vi "AddObject.vi"(1 "remote object ref":refnum<class "G#Object.lvclass">, 2 "proxy object ref":refnum<class "G#RemoteProxy.lvclass">, 3 "proxy class object ref":refnum<class "G#RemoteProxy.lvclass">, 5 "error in (no error)":errorcluster, 6 "full class name":string) -> (19 "error out":errorcluster)   [LabVIEW 2017, in "G#RemoteProxy.lvclass"]
doc: "Adds object to the local cache."
uses:
  G#RemoteProxy.lvclass
  G#Object/G#Object.lvclass
  C:/Program Files (x86)/National Instruments/LabVIEW 2017/vi.lib/addons/_AddQ/G#Object/G#Object.lvclass
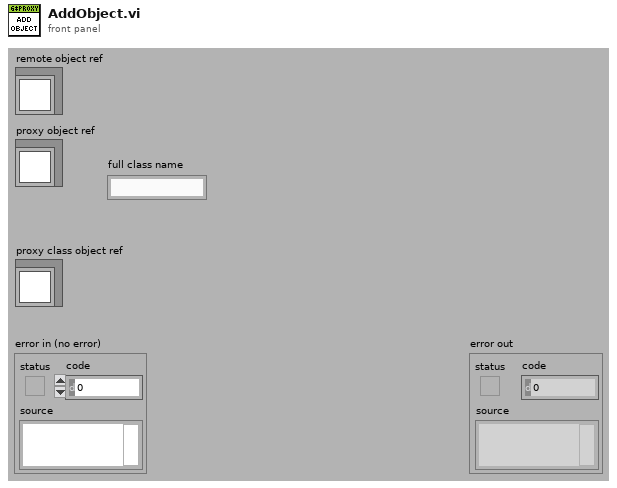
[diagram p1: front panel]
types:
  T1 = typedef "G#RemoteProxy.lvclass/ClassAttributesRef.ctl" = refnum<data-value>
  T2 = typedef "G#RemoteProxy.lvclass/ClassAttributesProxy.ctl" = cluster{"NoActiveProject":bool, "FullClassNames":string[], "FullClassPaths":path[], "RemoteRefs":refnum<class "G#Object.lvclass">[], "ProxyRefs":refnum<class "G#RemoteProxy.lvclass">[], "RemoteClassName":string[], "ProxyClassRefs":refnum<class "G#RemoteProxy.lvclass">[]}
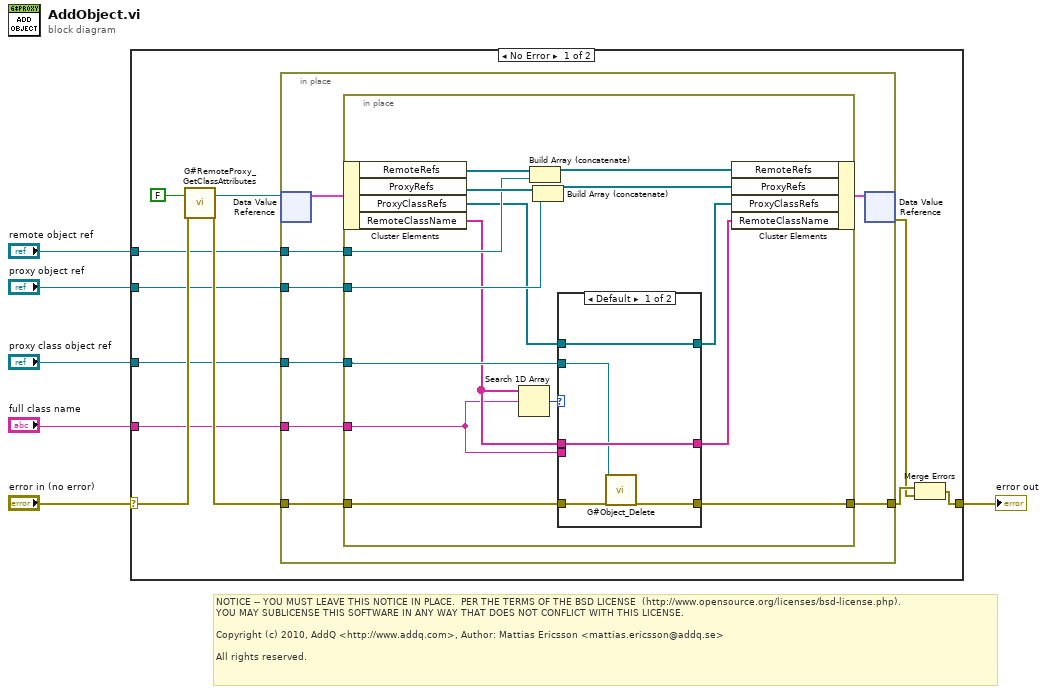
[diagram p0: block diagram]
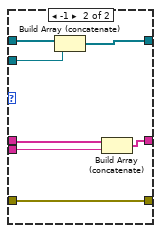
[diagram p2: hidden frame]
diagram:
  # "NOTICE -- YOU MUST LEAVE THIS NOTICE IN PLACE.  PER THE TERMS OF THE BSD LICENSE  (http://www.opensource.org/licenses/bsd-license.php).\nYOU MAY SUBLICENSE THIS SOFTWARE IN ANY WAY THAT DOES NOT CONFLICT WITH THIS LICENSE.\n\nCopyright (c) 2010, AddQ <http://www.addq.com>, Author: Mattias Ericsson <mattias.ericsson@addq.se>\n\nAll rights reserved."
  n1 = case shown="No Error" "error in (no error)" {
    selector: "error in (no error)" -> [w17 w53]
    tunnel: [w14 w53] -> w5
    tunnel: "remote object ref" -> [w10 _]
    tunnel: "proxy object ref" -> [w9 _]
    tunnel: "full class name" -> [w8 _]
    tunnel: "proxy class object ref" -> [w7 _]
    frame No Error {
      n2 = call "G#RemoteProxy_GetClassAttributes.vi"("return data? (T)"=FALSE ("return data"), "error in (no error)"=w17) -> ("class attributes ref"=w15:T1, "error out"=w16:errorcluster)  [unwired: 14 in, 2 out]
      n3 = in-place {
        in-place-border: w16 -> [w20]
        in-place-border: [w19] -> w12
        in-place-border: w10 -> [w23]
        in-place-border: w9 -> [w22]
        in-place-border: w8 -> [w21]
        in-place-border: w7 -> [w18]
        n4 = in-place-dvr #1(w15) -> (w24:T2)  [unwired: 1 out]
        n5 = in-place {
          in-place-border: w23 -> [w33]
          in-place-border: w22 -> [w36]
          in-place-border: w21 -> [w26]
          in-place-border: w20 -> [w34]
          in-place-border: [w29] -> w19
          in-place-border: w18 -> [w32]
          n6 = in-place-cluster #2(w24) -> ("RemoteRefs"=w40:refnum<class "G#Object.lvclass">[], "ProxyRefs"=w37:refnum<class "G#RemoteProxy.lvclass">[], "ProxyClassRefs"=w31:refnum<class "G#RemoteProxy.lvclass">[], "RemoteClassName"=w27:string[])
          n7 = Search 1D Array(1D array=w27, element=w26) -> (index of element=w35:i32)  [unwired: 1 in]
          n8 = Build Array (concatenate)(w40, w33) -> (w39:refnum<class "G#Object.lvclass">[])
          n9 = Build Array (concatenate)(w37, w36) -> (w38:refnum<class "G#RemoteProxy.lvclass">[])
          n10 = case shown="Default" w35 {
            tunnel: w34 -> [w43 w47]
            tunnel: w32 -> [w41 w51]
            tunnel: w27 -> [w44 w49]
            tunnel: w31 -> [w45 w52]
            tunnel: [w45 w50] -> w30
            tunnel: [w42 w47] -> w29
            tunnel: [w44 w48] -> w28
            tunnel: w26 -> [_ w46]
            frame Default {
              n11 = call "G#Object_Delete.vi"("reference in"=w41, "error in (no error)"=w43) -> ("error out"=w42:errorcluster)  [unwired: 16 in, 1 out]
            }
            frame -1 {
              n12 = Build Array (concatenate)(w52, w51) -> (w50:refnum<class "G#RemoteProxy.lvclass">[])
              n13 = Build Array (concatenate)(w49, w46) -> (w48:string[])
            }
          }
          n14 = in-place-cluster #2("RemoteRefs"=w39, "ProxyRefs"=w38, "ProxyClassRefs"=w30, "RemoteClassName"=w28) -> (w25:T2)
        }
        n15 = in-place-dvr #1(w25) -> (w11:errorcluster)  [unwired: 1 out]
      }
      n16 = Merge Errors(w12, w11) -> (w14:errorcluster)
    }
    frame Error {
    }
  }
  "error out" <- w5
